vi "Auto.vi"() -> ()   [LabVIEW 2020]
uses:
  Global_Variable/A131258.vi
  Global_Variable/Global.vi
  Database/Global1.vi
  <vilib>/addons/database/Connection.llb/DB Tools Open Connec (String).vi
  <vilib>/addons/database/Connection.llb/Conn Execute.vi
  <vilib>/addons/database/Recordset.llb/Rec Fetch Recordset Data (R).vi
  Global_Variable/A180648.vi
  Libraries/S7/S7.lvlib
  <userlib>/_MGI/1D Array/MGI Running Average/MGI Running Average(DBL[]).vi
  <vilib>/addons/database/NI_Database_API.lvlib
panel:
  out "试验项_Event":refnum<user-event>
  out "标尺_Event":refnum<user-event>
  in  "STEP":string
  out "NVH":bool=TRUE
  out "力特性逆向去程":bool
  out "力特性正向去程":bool
  out "力特性逆向回程":bool
  out "力特性正向回程":bool
  out "逆向空载正向初始化":bool
  out "锁紧/开启初始化":bool
  out "功能正向初始化":bool
  out "功能逆向初始化":bool
  out "空载逆向初始化":bool
  out "空载正向初始化":bool
  out "当前车速":i32
  out "试验项目":T1(tab)
  out "左工位曲线":cluster{dbl[], dbl[]}[](graph)
  out "右工位曲线":cluster{dbl[], dbl[]}[](graph)
  out "角度调节力试验":cluster{dbl[], dbl[]}[](graph)
  out "管柱保持力试验":cluster{dbl[], dbl[]}[](graph)
  out "锁紧/开启":cluster{dbl[], dbl[]}[](graph)
  out "逆向空载试验":cluster{dbl[], dbl[]}[](graph)
  out "振动2NHV-FFT":cluster{"f0":dbl, "df":dbl, "magnitude":dbl[]}[](graph)
  out "振动1NVH-FFT":cluster{"f0":dbl, "df":dbl, "magnitude":dbl[]}[](graph)
  in  "判定结果":bool[][](array[boolean])=[[TRUE]]
  # "."
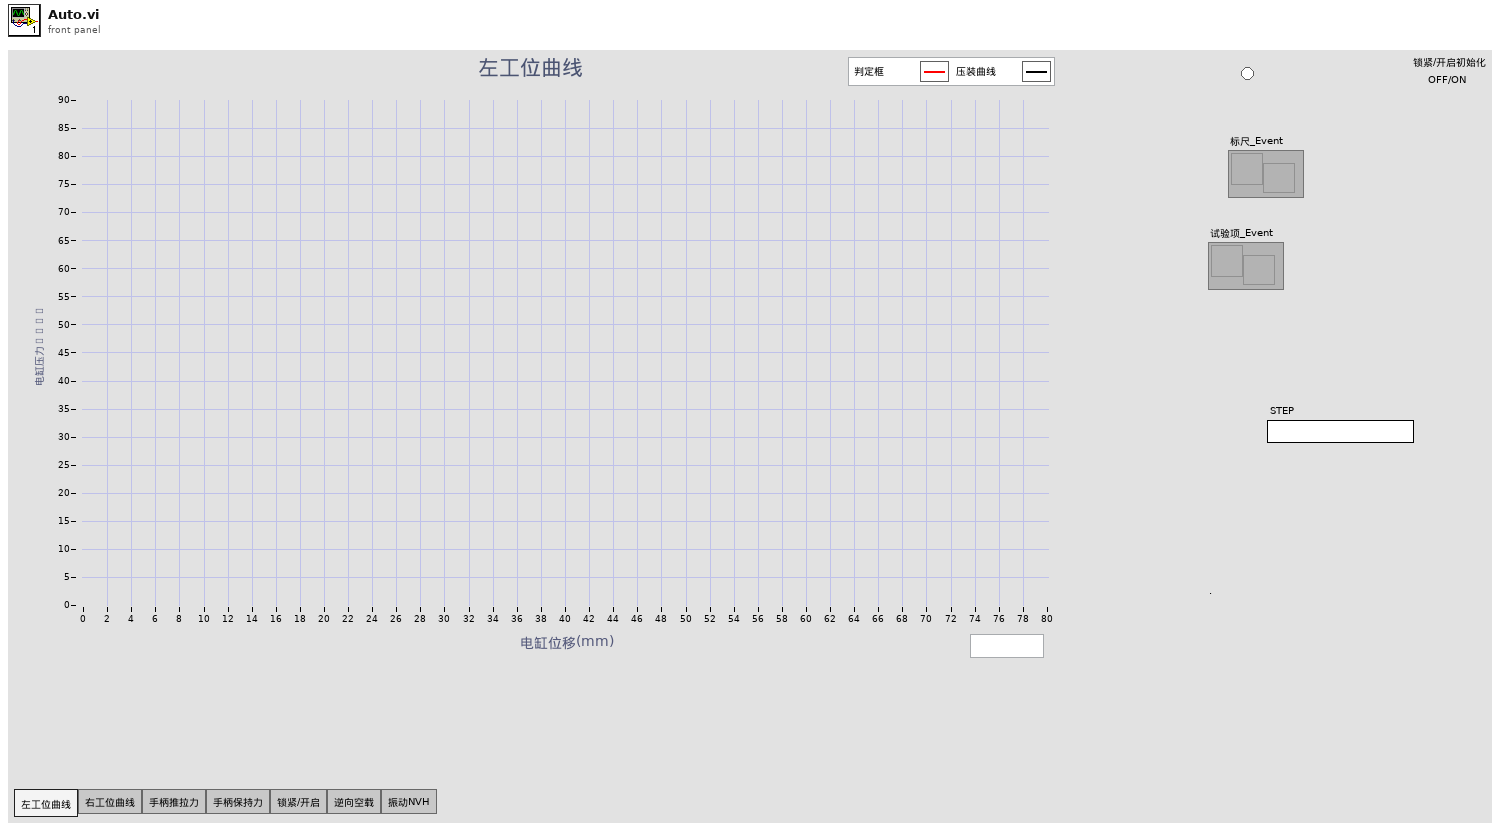
[diagram p1: front panel]
types:
  T1 = enum32{"左工位曲线", "右工位曲线", "手柄推拉力", "手柄保持力", "锁紧/开启", "逆向空载", "振动NVH"}
  T2 = typedef "NI_Database_API.lvlib/Conn ObjectReference.ctl" = refnum<k1>
  T3 = typedef "NI_Database_API.lvlib/Rec ObjectReference.ctl" = refnum<k1>
  T4 = cluster{"左工位最大压力 ":cluster{"单位":string, "下限":dbl, "上限":dbl}, "左工位最小压力":cluster{"单位":string, "下限":dbl, "上限":dbl}, "左工位最终压装位移":cluster{"单位":string, "下限":dbl, "上限":dbl}}
  T5 = cluster{"右工位最大压力 ":cluster{"单位":string, "下限":dbl, "上限":dbl}, "右工位最小压力":cluster{"单位":string, "下限":dbl, "上限":dbl}, "右工位最最终位移":cluster{"单位":string, "下限":dbl, "上限":dbl}}
  T6 = cluster{"X ":cluster{"单位":string, "下限":dbl, "上限":dbl}, "Y":cluster{"单位":string, "下限":dbl, "上限":dbl}}
  T7 = typedef "lveventtype.ctl" = enum32{"Null", "Timeout", "Annotation Menu Selection", "Annotation Menu Selection?", "App Instance Close", "App Instance Close?", "Autoscale Range Change", "Bookmark Info Change", "Cell Edit", "Cell Edit?", "Cursor Grab", "Cursor Grab?", "Cursor Menu Selection", "Cursor Menu Selection?", "Cursor Move", "Cursor Release", "Data Change", "Direction Change", "Display State Change", "Drag Ended", "Drag Enter", "Drag Leave", "Drag Over", "Drag Source Update", "Drag Starting", "Drag Starting?", "Drop", "Exec State Change", "Key Down", "Key Down?", "Key Repeat", "Key Repeat?", "Key Up", "Listbox Double Click", "Menu Activation?", "Menu Selection (App)", "Menu Selection? (App)", "Menu Selection (User)", "Mouse Down", "Mouse Down?", "Mouse Enter", "Mouse Leave", "Mouse Move", "Mouse Up", "Mouse Wheel", "NI Security User Change (App)", "Pane Size", "Panel Close", "Panel Close?", "Panel Resize", "Plot Attribute Change", "Scale Range Change", "Shortcut Menu Activation?", "Shortcut Menu Selection (App)", "Shortcut Menu Selection? (App)", "Shortcut Menu Selection (User)", "Tree Double Click", "Tree Drag", "Tree Drag?", "Tree Drop", "Tree Drop?", "Tree Item Close", "Tree Item Close?", "Tree Item Open", "Tree Item Open?", "User Event", "Value Change"}
  T8 = typedef "LVPoint32TypeDef.ctl" = cluster{"Horizontal":i32, "Vertical":i32}
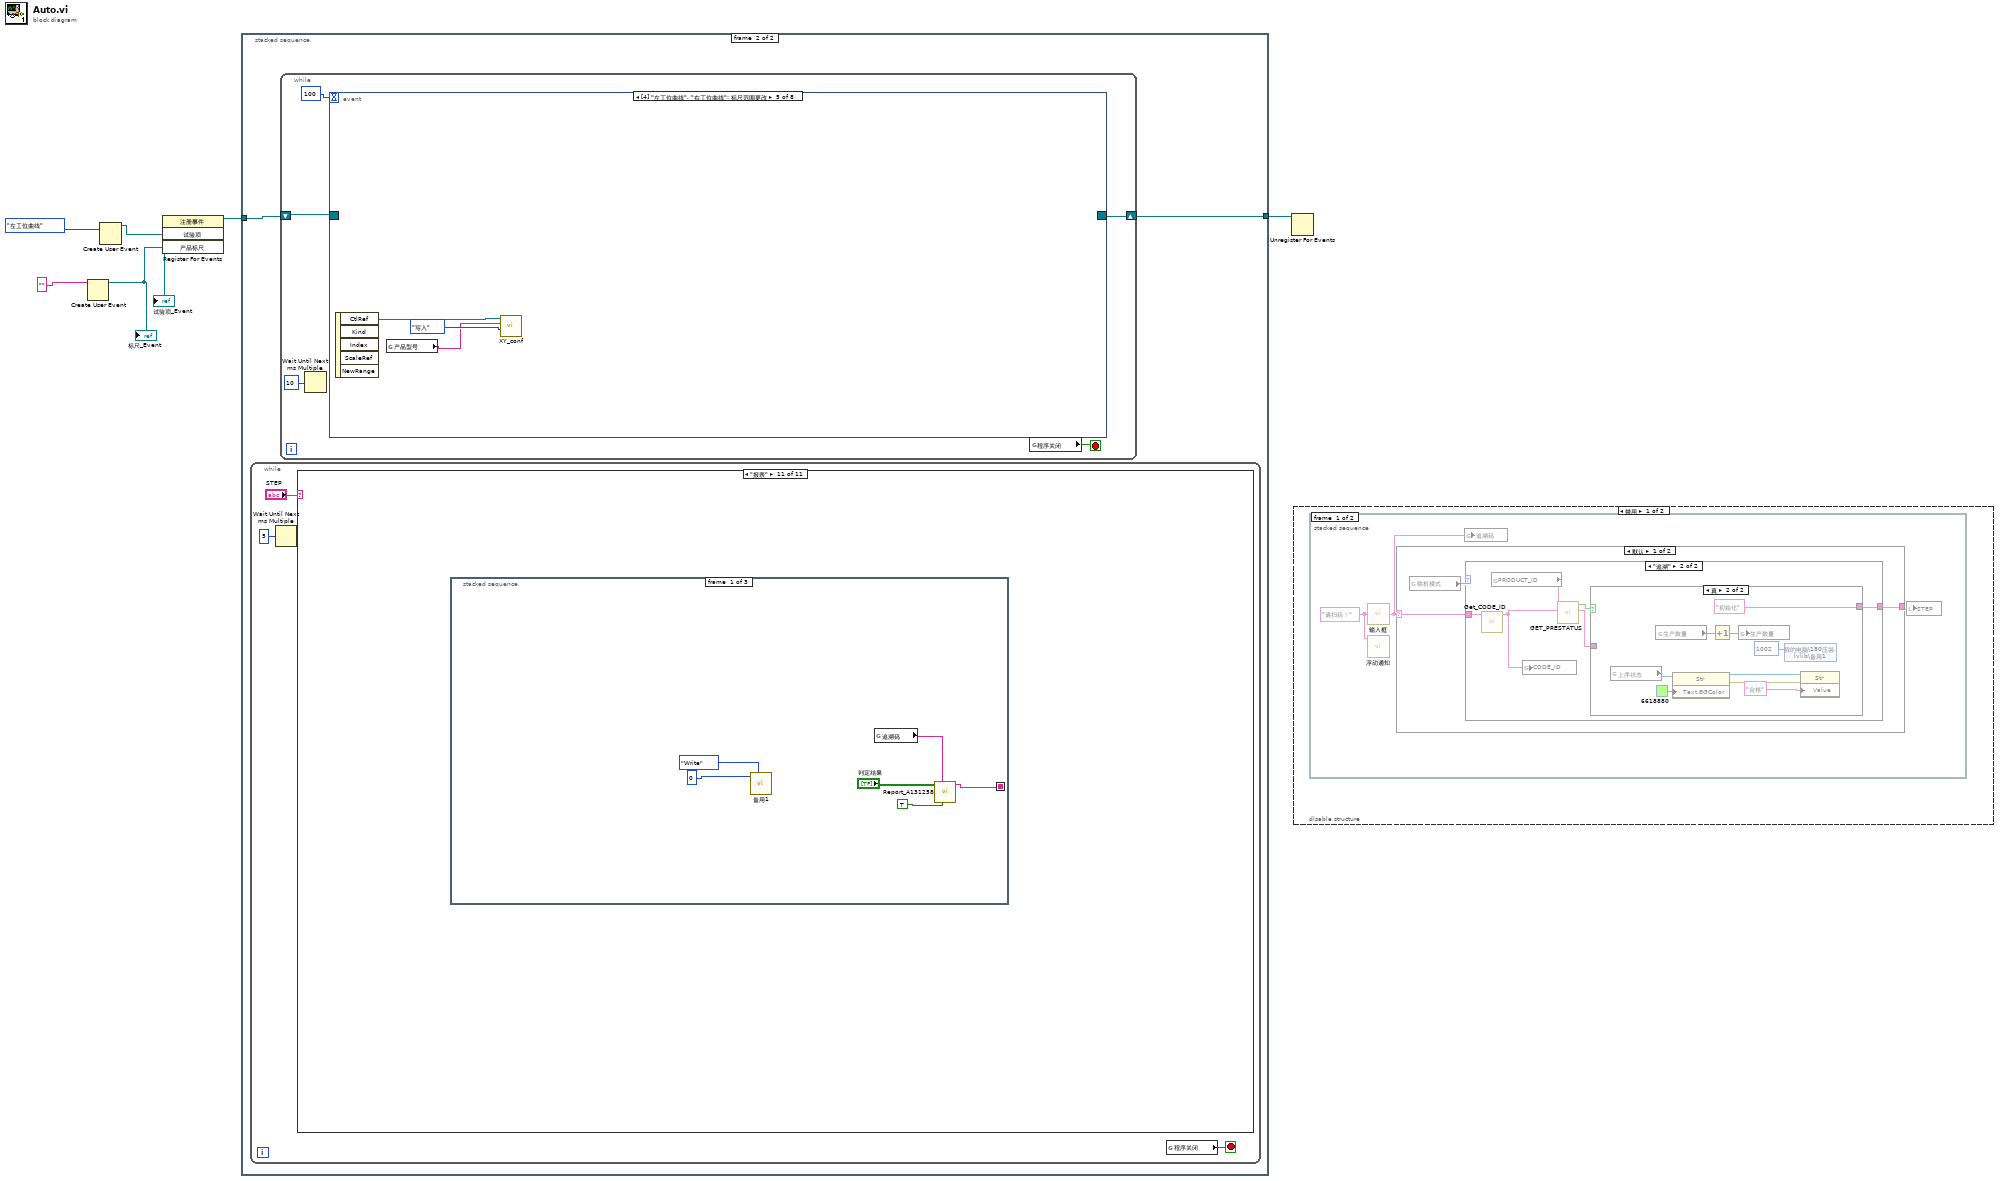
[diagram p0: block diagram]
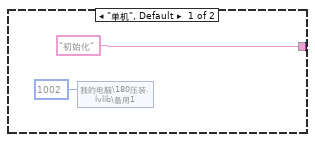
[diagram p2: hidden frame]
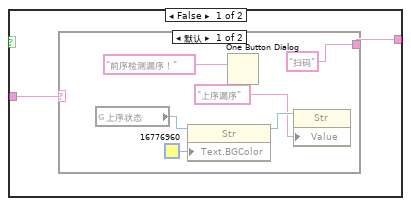
[diagram p3: hidden frame]
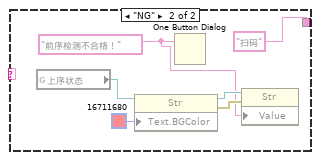
[diagram p4: hidden frame]
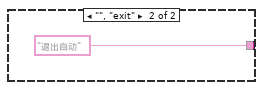
[diagram p5: hidden frame]
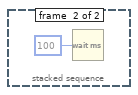
[diagram p6: hidden frame]
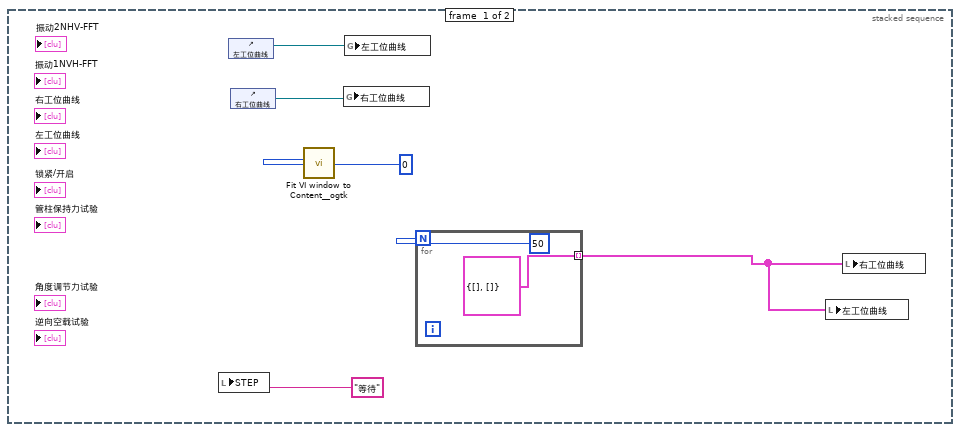
[diagram p8: hidden frame]
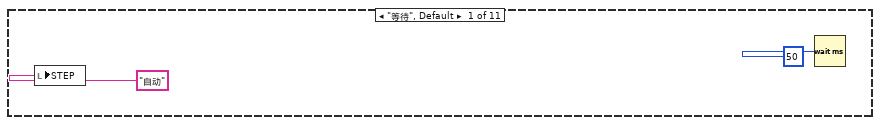
[diagram p9: hidden frame]
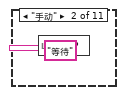
[diagram p10: hidden frame]
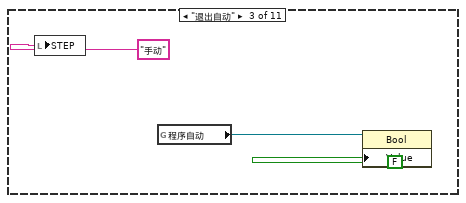
[diagram p11: hidden frame]
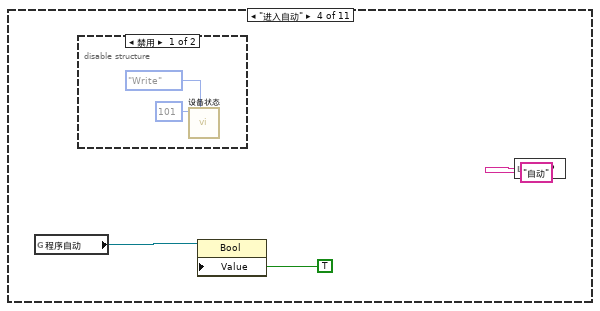
[diagram p12: hidden frame]
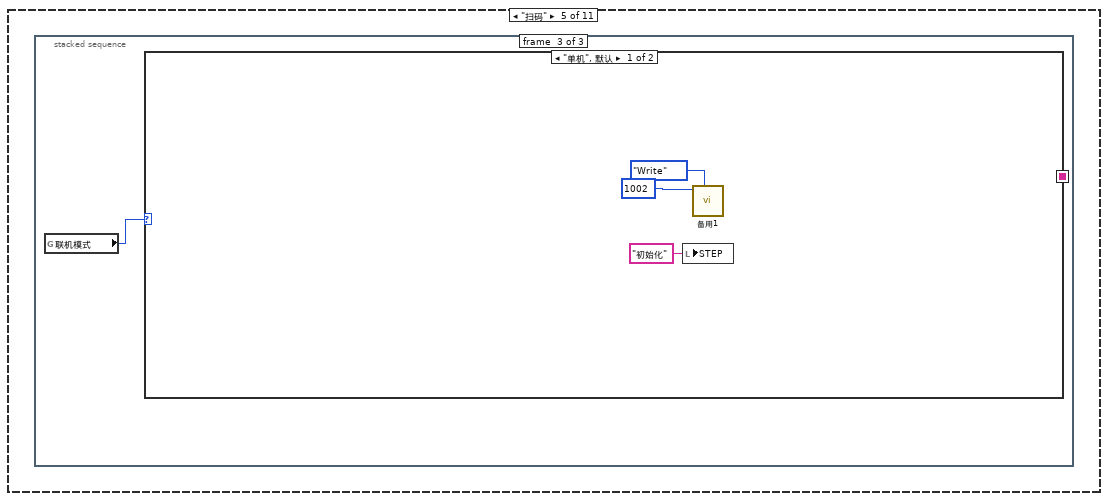
[diagram p14: hidden frame]
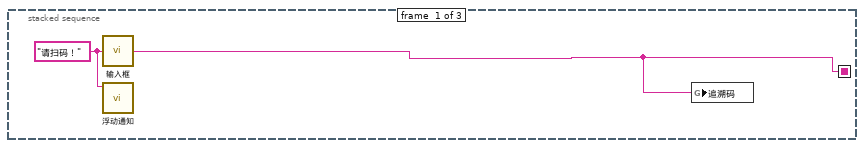
[diagram p15: hidden frame]
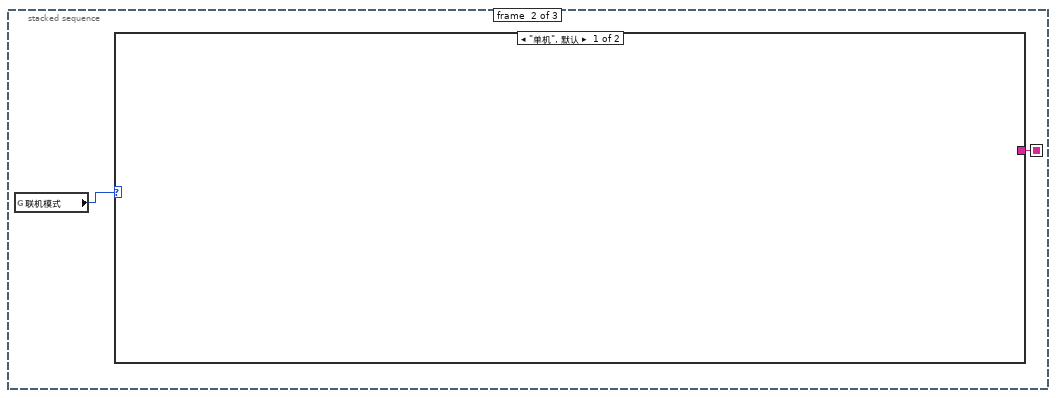
[diagram p16: hidden frame]
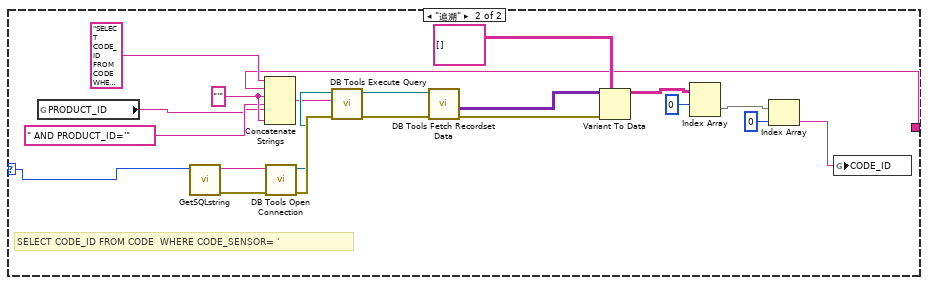
[diagram p17: hidden frame]
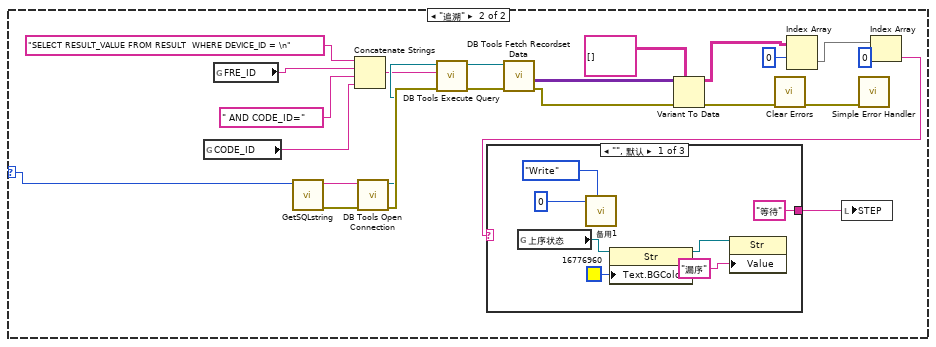
[diagram p18: hidden frame]
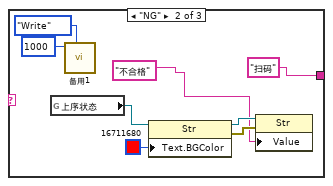
[diagram p19: hidden frame]
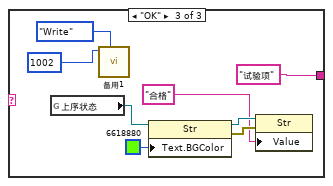
[diagram p20: hidden frame]
diagram:
  n1 = Create User Event(user event datatype="" ("产品标尺")) -> (user event=w4:refnum<user-event>)  [unwired: 1 in, 1 out]
  "标尺_Event" <- w4
  n2 = Create User Event(user event datatype=T1."左工位曲线" ("试验项")) -> (user event=w1:refnum<user-event>)  [unwired: 1 in, 1 out]
  "试验项_Event" <- w1
  n3 = register-events(w1, w4) -> (reference out=w5:refnum<event-registration>)  [unwired: 2 in, 1 out]
  n4 = stacked-sequence {
    tunnel: [_ w15] -> w6
    tunnel: w5 -> [_ w14]
    frame #0 {
      n5 = local write "STEP"("等待" ("STEP")) -> ()
      n6 = control-ref of="左工位曲线"() -> (w11:refnum<vi>)
      n7 = control-ref of="右工位曲线"() -> (w12:refnum<vi>)
      n8 = call "Fit VI window to Content__ogtk.vi"("border spacing (2 px)"=0) -> ()  [unwired: 5 in, 2 out]
      n9 = global write "A131258.vi" "右工位曲线"(w12) -> ()
      n10 = global write "A131258.vi" "左工位曲线"(w11) -> ()
      n11 = for {
        N: 50 -> [_]
        tunnel: [cluster{dbl[], dbl[]} {[], []}] -> w8 mode=indexing
      }
      n12 = local write "左工位曲线"(w8) -> ()
      n13 = local write "右工位曲线"(w8) -> ()
    }
    frame #1 {
      n14 = while {
        stop <- w18 stop-if-true
        n15 = Wait Until Next ms Multiple(millisecond multiple=u32 5 ("毫秒倍数")) -> ()  [unwired: 1 out]
        n16 = case shown="\"报表\"" "STEP" {
          frame "等待", Default {
            n17 = local write "STEP"("自动" ("STEP")) -> ()
            n18 = Wait (ms)(milliseconds to wait=u32 50 ("等待时间（毫秒）")) -> ()  [unwired: 1 out]
          }
          frame "手动" {
            n19 = local write "STEP"("等待" ("STEP")) -> ()
          }
          frame "退出自动" {
            n20 = local write "STEP"("手动" ("STEP")) -> ()
            n21 = global read "Global.vi" "程序自动"() -> (w23:refnum<vi>)
            n22 = property class="Bool"(reference=w23, "Value"=FALSE) -> ()  [unwired: 1 in, 2 out]
          }
          frame "进入自动" {
            n23 = global read "Global.vi" "程序自动"() -> (w26:refnum<vi>)
            n24 = disable-structure shown="禁用" {
              frame Disabled {
                n25 = call "设备状态.vi"("枚举"=enum16{"Read", "Write"}."Write", "Status_Write"=i16 101) -> ()  [unwired: 9 in, 1 out]
              }
              frame Enabled {
              }
            }
            n26 = property class="Bool"(reference=w26, "Value"=TRUE) -> ()  [unwired: 1 in, 2 out]
            n27 = local write "STEP"("自动" ("STEP")) -> ()
          }
          frame "扫码" {
            n28 = stacked-sequence {
              seq-local: [w30 _ _] -> [_ w33 _]
              frame #0 {
                w31 = "请扫码！" ("提示信息")
                n29 = call "输入框.vi"("提示信息"=w31) -> ("条形码输出"=w30:string)
                n30 = call "浮动通知.vi"("通知内容"=w31) -> ()  [unwired: 11 in]
                n31 = global write "Global.vi" "追溯码"(w30) -> ()
              }
              frame #1 {
                n32 = global read "Global1.vi" "联机模式"() -> (w32:enum16{"单机", "追溯"})
                n33 = case shown="\"单机\", 默认" w32 {
                  selector: w32 -> [_ w34]
                  tunnel: w33 -> [_ w37]
                  frame "单机", Default {
                  }
                  frame "追溯" {
                    w54 = "'" ("字符串")
                    # "SELECT CODE_ID FROM CODE  WHERE CODE_SENSOR= '"
                    n34 = global read "Global.vi" "PRODUCT_ID"() -> (w36:string)
                    n35 = call "GetSQLstring.vi"("联机模式"=w34) -> ("错误输出"=w40:errorcluster, "连接字符串"=w39:string)  [unwired: 9 in]
                    n36 = Concatenate Strings("SELECT CODE_ID FROM CODE  WHERE CODE_MAIN= '" ("table"), w37, w54, " AND PRODUCT_ID='" ("字符串"), w36, w54) -> (w41:string)
                    n37 = call-poly <vilib>:"DB Tools Open Connection.vi"("error in (no error)"=w40, "connection information"=w39) -> ("error out"=w46:errorcluster, "connection reference"=w45:T2)  [unwired: 6 in]
                    n38 = call-poly <vilib>:"DB Tools Execute Query.vi"("error in (no error)"=w46, "SQL query"=w41, "connection reference"=w45) -> ("error out"=w43:errorcluster, "recordset reference"=w42:T3)  [unwired: 5 in]
                    n39 = call-poly <vilib>:"DB Tools Fetch Recordset Data.vi"("error in (no error)"=w43, "recordset reference"=w42) -> ("error out"=w48:errorcluster, "recordset data"=w44:variant[][])  [unwired: 3 in, 1 out]
                    n40 = Variant To Data(error in=w48, type=string[][] [], Variant=w44) -> (data=w49:string[][])  [unwired: 1 out]
                    n41 = Index Array(array=w49, index (row)=0 ("索引 (行)")) -> (element=w51:string[])  [unwired: 1 in]
                    n42 = Index Array(array=w51, index=0 ("索引 (行)")) -> (element=w35:string)
                    n43 = global write "Global.vi" "CODE_ID"(w35) -> ()
                  }
                }
              }
              frame #2 {
                n44 = global read "Global1.vi" "联机模式"() -> (w55:enum16{"单机", "追溯"})
                n45 = case shown="\"单机\", 默认" w55 {
                  selector: w55 -> [_ w59]
                  frame "单机", Default {
                    n46 = local write "STEP"("初始化" ("STEP")) -> ()
                    n47 = call "备用1.vi"("枚举"=enum16{"Read", "Write"}."Write", "Status_Write"=u16 1002 ("备用1")) -> ()  [unwired: 9 in, 1 out]
                  }
                  frame "追溯" {
                    n48 = global read "Global.vi" "CODE_ID"() -> (w62:string)
                    n49 = global read "Global.vi" "FRE_ID"() -> (w63:string)
                    n50 = call "GetSQLstring.vi"("联机模式"=w59) -> ("错误输出"=w65:errorcluster, "连接字符串"=w64:string)  [unwired: 9 in]
                    n51 = Concatenate Strings("SELECT RESULT_VALUE FROM RESULT  WHERE DEVICE_ID = \n" ("table"), w63, " AND CODE_ID=" ("字符串"), w62) -> (w66:string)
                    n52 = call-poly <vilib>:"DB Tools Open Connection.vi"("error in (no error)"=w65, "connection information"=w64) -> ("error out"=w72:errorcluster, "connection reference"=w71:T2)  [unwired: 6 in]
                    n53 = call-poly <vilib>:"DB Tools Execute Query.vi"("error in (no error)"=w72, "SQL query"=w66, "connection reference"=w71) -> ("error out"=w68:errorcluster, "recordset reference"=w67:T3)  [unwired: 5 in]
                    n54 = call-poly <vilib>:"DB Tools Fetch Recordset Data.vi"("error in (no error)"=w68, "recordset reference"=w67) -> ("error out"=w74:errorcluster, "recordset data"=w69:variant[][])  [unwired: 3 in, 1 out]
                    n55 = Variant To Data(error in=w74, type=string[][] [], Variant=w69) -> (data=w78:string[][], error out=w79:errorcluster)
                    n56 = call <vilib>:"Clear Errors.vi"("error in (no error)"=w79) -> ("error out"=w80:errorcluster)  [unwired: 5 in, 1 out]
                    n57 = Index Array(array=w78, index (row)=0 ("索引 (行)")) -> (element=w76:string[])  [unwired: 1 in]
                    n58 = call <vilib>:"Simple Error Handler.vi"("error in (no error)"=w80) -> ()  [unwired: 4 in, 5 out]
                    n59 = Index Array(array=w76, index=0 ("索引 (行)")) -> (element=w61:string)
                    n60 = case shown="\"\", 默认" w61 {
                      tunnel: ["等待" ("State(s) in Front (\"\")") "扫码" ("State(s) in Front (\"\")") "试验项" ("State(s) in Front (\"\")")] -> w60
                      frame "", Default {
                        n61 = global read "Global.vi" "上序状态"() -> (w85:refnum<vi>)
                        n62 = call "备用1.vi"("枚举"=enum16{"Read", "Write"}."Write", "Status_Write"=u16 0 ("备用1")) -> ()  [unwired: 9 in, 1 out]
                        n63 = property class="Str"(reference=w85, "Text.BGColor"=u32 16776960 ("文本.文本颜色:背景色")) -> (reference out=w86:refnum<vi>)  [unwired: 1 in, 1 out]
                        n64 = property class="Str"(reference=w86, "Value"="漏序" ("上序状态")) -> ()  [unwired: 1 in, 2 out]
                      }
                      frame "NG" {
                        n65 = global read "Global.vi" "上序状态"() -> (w92:refnum<vi>)
                        n66 = call "备用1.vi"("枚举"=enum16{"Read", "Write"}."Write", "Status_Write"=i16 1000) -> ()  [unwired: 9 in, 1 out]
                        n67 = property class="Str"(reference=w92, "Text.BGColor"=u32 16711680 ("文本.文本颜色:背景色")) -> (reference out=w95:refnum<vi>, error out=w94:errorcluster)  [unwired: 1 in]
                        n68 = property class="Str"(reference=w95, error in=w94, "Value"="不合格" ("消息")) -> ()  [unwired: 2 out]
                      }
                      frame "OK" {
                        n69 = global read "Global.vi" "上序状态"() -> (w100:refnum<vi>)
                        n70 = call "备用1.vi"("枚举"=enum16{"Read", "Write"}."Write", "Status_Write"=u16 1002 ("备用1")) -> ()  [unwired: 9 in, 1 out]
                        n71 = property class="Str"(reference=w100, "Text.BGColor"=u32 6618880 ("文本.文本颜色:背景色")) -> (reference out=w103:refnum<vi>, error out=w102:errorcluster)  [unwired: 1 in]
                        n72 = property class="Str"(reference=w103, error in=w102, "Value"="合格" ("消息")) -> ()  [unwired: 2 out]
                      }
                    }
                    n73 = local write "STEP"(w60) -> ()
                  }
                }
              }
            }
          }
          frame "等待启动" {
            n74 = local write "STEP"("等待" ("STEP")) -> ()
          }
          frame "初始化" {
            n75 = stacked-sequence {
              frame #0 {
                w106 = 0 ("当前车速")
                n76 = local write "判定结果"(bool[][] [] ("判定结果")) -> ()
                n77 = global write "Global.vi" "右判定长度"(w106) -> ()
                n78 = global write "Global.vi" "左判定长度"(w106) -> ()
                "当前车速" <- w106
              }
              frame #1 {
                w111 = TRUE
                n79 = global read "Global.vi" "试验项目"() -> (w110:bool[])
                n80 = Index Array(array=w110, index=4 ("索引")) -> (element=w108:bool)
                n81 = case shown="假" w108 {
                  frame False {
                    n82 = local write "锁紧/开启初始化"(FALSE ("锁紧/开启初始化")) -> ()
                  }
                  frame True {
                    "锁紧/开启初始化" <- TRUE ("锁紧/开启初始化")
                  }
                }
                "逆向空载正向初始化" <- w111
                "空载正向初始化" <- w111
                "空载逆向初始化" <- w111
                "功能正向初始化" <- w111
                "功能逆向初始化" <- w111
                "力特性逆向去程" <- w111
                "力特性正向去程" <- w111
                "力特性逆向回程" <- w111
                "力特性正向回程" <- w111
              }
              frame #2 {
                n83 = for {
                  N: 50 -> [_]
                  tunnel: [cluster{dbl[], dbl[]} {[], []}] -> w115 mode=indexing
                  tunnel: [cluster{"f0":dbl, "df":dbl, "magnitude":dbl[]} {"f0"=0.0, "df"=0.0, "magnitude"=[]} ("power spectrum [dB EU]")] -> w114 mode=indexing
                }
                n84 = local write "角度调节力试验"(w115) -> ()
                n85 = local write "管柱保持力试验"(w115) -> ()
                n86 = local write "逆向空载试验"(w115) -> ()
                n87 = local write "锁紧/开启"(w115) -> ()
                n88 = local write "左工位曲线"(w115) -> ()
                n89 = local write "右工位曲线"(w115) -> ()
                n90 = local write "振动2NHV-FFT"(w114) -> ()
                n91 = local write "振动1NVH-FFT"(w114) -> ()
              }
              frame #3 {
                w120 = -2
                n92 = global read "Global.vi" "Result"() -> (w122:refnum<vi>)
                n93 = Bundle(w120, w120) -> (w119:cluster{i32, i32})  [unwired: 1 in]
                n94 = property class="Tbl"(reference=w122, "Value"=string[][] []) -> (reference out=w125:refnum<vi>, error out=w126:errorcluster)  [unwired: 1 in]
                n95 = property class="Tbl"(reference=w122, "Active Cell"=w119, "Cell BG Color"=u32 16777216 ("活动单元格:单元格背景色")) -> ()  [unwired: 1 in, 2 out]
                n96 = property class="Tbl"(reference=w125, error in=w126, "Row Headers[]"=string[] [] ("列首字符串[]")) -> ()  [unwired: 2 out]
              }
              frame #4 {
                n97 = global read "A131258.vi" "LED-左工位"() -> (w128:refnum<vi>)
                n98 = global read "A131258.vi" "LED-右工位"() -> (w127:refnum<vi>)
                n99 = Build Array(w128, w127) -> (w129:refnum<vi>[])
                n100 = for {
                  tunnel: w129 -> [w130] mode=indexing
                  n101 = property class="Bool"(reference=w130, "Colors [4]"=cluster{u32, u32}[] [{12369084, 12369084}] ("颜色[4]")) -> ()  [unwired: 1 in, 2 out]
                }
              }
              frame #5 {
                n102 = global write "Global.vi" "当前试验项"(enum16{"左工位", "右工位", "完成"}."左工位" ("当前试验项")) -> ()
                n103 = local write "STEP"("试验项" ("STEP")) -> ()
              }
            }
          }
          frame "试验项" {
            n104 = global read "Global.vi" "当前试验项"() -> (w134:enum16{"左工位", "右工位", "完成"})
            n105 = case shown="\"完成\"" w134 {
              selector: w134 -> [w136 _]
              tunnel: [w139 "报表" ("STEP")] -> w135
              frame "左工位", Default {
                n106 = global read "Global.vi" "试验项目"() -> (w137:bool[])
                n107 = Index Array(array=w137, index=w136) -> (element=w138:bool)
                n108 = case shown="真" w138 {
                  selector: w138 -> [_ w146]
                  tunnel: ["试验项" ("字符串") w147] -> w139
                  tunnel: w136 -> [_ w148]
                  frame False {
                    n109 = global read "Global.vi" "当前试验项"() -> (w141:enum16{"左工位", "右工位", "完成"})
                    n110 = Increment(x=w141) -> (x+1=w140:enum16{"左工位", "右工位", "完成"})
                    n111 = local read "判定结果"() -> (w142:bool[][])
                    n112 = global write "Global.vi" "当前试验项"(w140) -> ()
                    n113 = Build Array (concatenate)(w142, bool[] [FALSE] ("判定结果")) -> (w143:bool[][])
                    n114 = local write "判定结果"(w143) -> ()
                  }
                  frame True {
                    n115 = case shown="\"右工位\"" w148 {
                      tunnel: [w163 "等待" ("STEP") "试验项" ("STEP")] -> w147
                      tunnel: w146 -> [_ _ _]
                      frame "左工位", Default {
                        w156 = -2
                        n116 = global read "Global.vi" "Result"() -> (w158:refnum<vi>)
                        n117 = global write "Global.vi" "左判定长度"(0 ("左判定长度")) -> ()
                        n118 = property class="Tbl"(reference=w158, "Value"=string[][] []) -> (reference out=w161:refnum<vi>, error out=w162:errorcluster)  [unwired: 1 in]
                        n119 = local write "判定结果"(bool[][] [[FALSE]] ("判定结果")) -> ()
                        n120 = Bundle(w156, w156) -> (w155:cluster{i32, i32})  [unwired: 1 in]
                        n121 = global read "Global.vi" "复选框"() -> (w149:bool)
                        n122 = property class="Tbl"(reference=w161, error in=w162, "Row Headers[]"=string[] [] ("列首字符串[]")) -> ()  [unwired: 2 out]
                        n123 = property class="Tbl"(reference=w158, "Active Cell"=w155, "Cell BG Color"=u32 16777216 ("活动单元格:单元格背景色")) -> ()  [unwired: 1 in, 2 out]
                        n124 = global read "A131258.vi" "LED-右工位"() -> (w153:refnum<vi>)
                        n125 = global read "A131258.vi" "LED-左工位"() -> (w154:refnum<vi>)
                        n126 = case shown="假" w149 {
                          tunnel: ["试验项" ("STEP") "等待" ("STEP")] -> w163
                          frame False {
                            n127 = global read "Global.vi" "当前试验项"() -> (w165:enum16{"左工位", "右工位", "完成"})
                            n128 = Increment(x=w165) -> (x+1=w164:enum16{"左工位", "右工位", "完成"})
                            n129 = global write "Global.vi" "当前试验项"(w164) -> ()
                          }
                          frame True {
                            n130 = property on="试验项目" class="TabCtl (严格)"("Val(Sgnl)"=T1."左工位曲线" ("值(信号)")) -> ()  [unwired: 2 in, 2 out]
                            n131 = call "浮动通知.vi"("通知内容"="左工位压装") -> ()  [unwired: 11 in]
                          }
                        }
                        n132 = Build Array(w154, w153) -> (w152:refnum<vi>[])
                        n133 = for {
                          tunnel: w152 -> [w171] mode=indexing
                          n134 = property class="Bool"(reference=w171, "Colors [4]"=cluster{u32, u32}[] [{12369084, 12369084}] ("颜色[4]")) -> ()  [unwired: 1 in, 2 out]
                        }
                      }
                      frame "右工位" {
                        n135 = global read "Global.vi" "试验项目"() -> (w174:bool[])
                        n136 = property on="试验项目" class="TabCtl (严格)"("Val(Sgnl)"=T1."右工位曲线" ("值(信号)")) -> ()  [unwired: 2 in, 2 out]
                        n137 = call "浮动通知.vi"("通知内容"="右工位压装") -> ()  [unwired: 11 in]
                        n138 = Index Array(array=w174, index=0 ("索引")) -> (element=w173:bool)
                        n139 = case shown="假" w173 {
                          frame False {
                            w184 = -2
                            n140 = global read "Global.vi" "Result"() -> (w186:refnum<vi>)
                            n141 = Bundle(w184, w184) -> (w183:cluster{i32, i32})  [unwired: 1 in]
                            n142 = global write "Global.vi" "左判定长度"(0 ("左判定长度")) -> ()
                            n143 = property class="Tbl"(reference=w186, "Value"=string[][] []) -> (reference out=w189:refnum<vi>, error out=w190:errorcluster)  [unwired: 1 in]
                            n144 = property class="Tbl"(reference=w186, "Active Cell"=w183, "Cell BG Color"=u32 16777216 ("活动单元格:单元格背景色")) -> ()  [unwired: 1 in, 2 out]
                            n145 = property class="Tbl"(reference=w189, error in=w190, "Row Headers[]"=string[] [] ("列首字符串[]")) -> ()  [unwired: 2 out]
                            n146 = global read "A131258.vi" "LED-右工位"() -> (w181:refnum<vi>)
                            n147 = global read "A131258.vi" "LED-左工位"() -> (w182:refnum<vi>)
                            n148 = local write "判定结果"(bool[][] [[FALSE]] ("判定结果")) -> ()
                            n149 = Build Array(w182, w181) -> (w180:refnum<vi>[])
                            n150 = for {
                              tunnel: w180 -> [w192] mode=indexing
                              n151 = property class="Bool"(reference=w192, "Colors [4]"=cluster{u32, u32}[] [{12369084, 12369084}] ("颜色[4]")) -> ()  [unwired: 1 in, 2 out]
                            }
                          }
                          frame True {
                          }
                        }
                      }
                      frame "完成" {
                        n152 = call "浮动通知.vi"("通知内容"="压装完成") -> ()  [unwired: 11 in]
                      }
                    }
                  }
                }
              }
              frame "完成" {
                n153 = Wait (ms)(milliseconds to wait=u32 200 ("等待时间（毫秒）")) -> ()  [unwired: 1 out]
              }
            }
            n154 = local write "STEP"(w135) -> ()
          }
          frame "判定" {
            n155 = stacked-sequence {
              frame #0 {
                n156 = global read "Global.vi" "当前试验项"() -> (w197:enum16{"左工位", "右工位", "完成"})
                n157 = case shown="\"左工位\"" w197 {
                  frame "完成", Default {
                  }
                  frame "左工位" {
                    n158 = global read "Global.vi" "左工位判定参数"() -> (w200:T4)
                    n159 = global read "A131258.vi" "LED-左工位"() -> (w198:refnum<vi>)
                    n160 = local read "左工位曲线"() -> (w210:cluster{dbl[], dbl[]}[])
                    n161 = global read "Global.vi" "Result"() -> (w209:refnum<vi>)
                    n162 = call "左工位判定.vi"("Result"=w209, "左工位判定"=w200, "XY曲线"=w210) -> ("大小"=w199:i32, "OK？"=w201:bool)  [unwired: 7 in]
                    n163 = Select(t=cluster{u32, u32}[] [{6618880, 6618880}, {6618880, 6618880}, {6618880, 6618880}, {6618880, 6618880}] ("颜色[4]"), s=w201, f=cluster{u32, u32}[] [{16711680, 16711680}, {16711680, 16711680}, {16711680, 16711680}, {16711680, 16711680}] ("颜色[4]")) -> (s? t:f=w206:cluster{u32, u32}[])
                    n164 = property class="Bool"(reference=w198, "Colors [4]"=w206) -> ()  [unwired: 1 in, 2 out]
                    n165 = local read "判定结果"() -> (w202:bool[][])
                    n166 = case shown="假" w201 {
                      frame False {
                        w211 = 4 items=["OK", "OKCancel", "AbortRetryIgnore", "YesNoCancel", "YesNo", "RetryCancel"] ("buttons")
                        w213 = 64 items=["None"=0, "Hand, Error, Stop"=16, "Question"=32, "Exclamation, Warning"=48, "Asterisk, Information"=64] ("icon")
                        n167 = call "信息框（标题、文本、图标）.vi"("icon"=w213, "buttons"=w211, "caption"="不合格", "text"="压装不合格是否进行下工位压装" ("消息")) -> ("按钮输出"=w212:i32)  [unwired: 6 in, 1 out]
                        n168 = case shown="7" w212 {
                          frame 6, Default {
                            n169 = local write "STEP"("报表" ("STEP")) -> ()
                          }
                          frame 7 {
                            n170 = global read "Global.vi" "当前试验项"() -> (w219:enum16{"左工位", "右工位", "完成"})
                            n171 = Increment(x=w219) -> (x+1=w220:enum16{"左工位", "右工位", "完成"})
                            n172 = global write "Global.vi" "当前试验项"(w220) -> ()
                          }
                        }
                        n173 = call "合格状态.vi"("枚举"=enum16{"Read", "Write"}."Write", "Status_Write"=i16 2) -> ()  [unwired: 9 in, 1 out]
                      }
                      frame True {
                        n174 = call "合格状态.vi"("枚举"=enum16{"Read", "Write"}."Write", "Status_Write"=i16 1) -> ()  [unwired: 9 in, 1 out]
                      }
                    }
                    n175 = Build Array(TRUE, w201) -> (w205:bool[])
                    n176 = Build Array (concatenate)(w202, w205) -> (w203:bool[][])
                    n177 = local write "判定结果"(w203) -> ()
                    n178 = global write "Global.vi" "左判定长度"(w199) -> ()
                  }
                  frame "右工位" {
                    n179 = global read "Global.vi" "右工位判定参数"() -> (w223:T5)
                    n180 = local read "右工位曲线"() -> (w236:cluster{dbl[], dbl[]}[])
                    n181 = global read "A131258.vi" "LED-右工位"() -> (w225:refnum<vi>)
                    n182 = global read "Global.vi" "Result"() -> (w235:refnum<vi>)
                    n183 = call "右工位判定.vi"("Result"=w235, "右工位判定"=w223, "XY曲线"=w236) -> ("大小"=w224:i32, "OK？"=w226:bool)  [unwired: 7 in]
                    n184 = Select(t=cluster{u32, u32}[] [{6618880, 6618880}, {6618880, 6618880}, {6618880, 6618880}, {6618880, 6618880}] ("颜色[4]"), s=w226, f=cluster{u32, u32}[] [{16711680, 16711680}, {16711680, 16711680}, {16711680, 16711680}, {16711680, 16711680}] ("颜色[4]")) -> (s? t:f=w232:cluster{u32, u32}[])
                    n185 = property class="Bool"(reference=w225, "Colors [4]"=w232) -> ()  [unwired: 1 in, 2 out]
                    n186 = local read "判定结果"() -> (w228:bool[][])
                    n187 = Build Array(TRUE, w226) -> (w231:bool[])
                    n188 = global write "Global.vi" "右判定长度"(w224) -> ()
                    n189 = Build Array (concatenate)(w228, w231) -> (w229:bool[][])
                    n190 = case shown="真" w226 {
                      frame False {
                        n191 = call "合格状态.vi"("枚举"=enum16{"Read", "Write"}."Write", "Status_Write"=i16 2) -> ()  [unwired: 9 in, 1 out]
                      }
                      frame True {
                        n192 = call "合格状态.vi"("枚举"=enum16{"Read", "Write"}."Write", "Status_Write"=i16 1) -> ()  [unwired: 9 in, 1 out]
                      }
                    }
                    n193 = local write "判定结果"(w229) -> ()
                    "NVH" <- TRUE
                  }
                }
              }
              frame #1 {
                n194 = global read "Global.vi" "当前试验项"() -> (w243:enum16{"左工位", "右工位", "完成"})
                n195 = Increment(x=w243) -> (x+1=w242:enum16{"左工位", "右工位", "完成"})
                n196 = local write "STEP"("试验项" ("STEP")) -> ()
                n197 = Wait (ms)(milliseconds to wait=u32 500 ("等待时间（毫秒）")) -> ()  [unwired: 1 out]
                n198 = global write "Global.vi" "当前试验项"(w242) -> ()
              }
            }
          }
          frame "自动" {
            n199 = call "备用1.vi"("枚举"=enum16{"Read", "Write"}."Read") -> ("Status_Read"=w246:i16)  [unwired: 10 in]
            n200 = case shown="1000" w246 {
              frame 0, Default {
              }
              frame 1 {
                n201 = call "备用2.vi"("枚举"=enum16{"Read", "Write"}."Read") -> ("Status_Read"=w250:i16)  [unwired: 10 in]
                n202 = call "传感器数据.vi"() -> ("电缸位移"=w248:sgl, "电缸自带压力"=w247:sgl)  [unwired: 7 in, 3 out]
                n203 = case shown="2" w250 {
                  tunnel: w248 -> [_ w252 w261]
                  tunnel: w247 -> [_ w251 w260]
                  frame 0, Default {
                  }
                  frame 1 {
                    n204 = control-ref of="左工位曲线"() -> (w256:refnum<vi>)
                    n205 = call "曲线采集.vi"("曲线引用"=w256, "曲线索引"=1, "X"=w252, "Y"=w251) -> ("错误输出"=w254:errorcluster)  [unwired: 10 in, 1 out]
                    n206 = Unbundle By Name(w254) -> ("status"=w253:bool)
                    n207 = local read "空载正向初始化"() -> (w257:bool)
                    n208 = local write "空载正向初始化"(w253) -> ()
                    n209 = disable-structure shown="禁用" {
                      disable-tunnel: w257 -> [w259 _]
                      frame Disabled {
                        w258 = 2 ("Averaging Size")
                        n210 = call-poly <userlib>:"MGI Running Average.vi"("Averaging Size"=w258, "Initialize? (F)"=w259) -> ()  [unwired: 9 in, 1 out]
                        n211 = call-poly <userlib>:"MGI Running Average.vi"("Averaging Size"=w258, "Initialize? (F)"=w259) -> ()  [unwired: 9 in, 1 out]
                      }
                      frame Enabled {
                      }
                    }
                  }
                  frame 2 {
                    n212 = control-ref of="右工位曲线"() -> (w265:refnum<vi>)
                    n213 = call "曲线采集.vi"("曲线引用"=w265, "曲线索引"=1, "X"=w261, "Y"=w260) -> ("错误输出"=w263:errorcluster)  [unwired: 10 in, 1 out]
                    n214 = Unbundle By Name(w263) -> ("status"=w262:bool)
                    n215 = local read "空载正向初始化"() -> (w266:bool)
                    n216 = local write "空载正向初始化"(w262) -> ()
                    n217 = disable-structure shown="禁用" {
                      disable-tunnel: w266 -> [w268 _]
                      frame Disabled {
                        w267 = 2 ("Averaging Size")
                        n218 = call-poly <userlib>:"MGI Running Average.vi"("Averaging Size"=w267, "Initialize? (F)"=w268) -> ()  [unwired: 9 in, 1 out]
                        n219 = call-poly <userlib>:"MGI Running Average.vi"("Averaging Size"=w267, "Initialize? (F)"=w268) -> ()  [unwired: 9 in, 1 out]
                      }
                      frame Enabled {
                      }
                    }
                  }
                }
              }
              frame 2 {
                n220 = flat-sequence {
                  frame #0 {
                    n221 = Wait (ms)(milliseconds to wait=u32 50 ("等待时间（毫秒）")) -> ()  [unwired: 1 out]
                    n222 = call "备用1.vi"("枚举"=enum16{"Read", "Write"}."Write", "Status_Write"=u16 0 ("备用1")) -> ()  [unwired: 9 in, 1 out]
                  }
                  frame #1 {
                    n223 = local write "STEP"("判定" ("STEP")) -> ()
                  }
                }
              }
              frame 3 {
                n224 = local write "STEP"("判定" ("STEP")) -> ()
                n225 = call "备用1.vi"("枚举"=enum16{"Read", "Write"}."Write", "Status_Write"=u16 0 ("备用1")) -> ()  [unwired: 9 in, 1 out]
              }
              frame 100 {
                n226 = global read "Global.vi" "当前试验项"() -> (w276:enum16{"左工位", "右工位", "完成"})
                n227 = case shown="\"左工位\"" w276 {
                  frame "完成", Default {
                  }
                  frame "左工位" {
                    n228 = stacked-sequence {
                      frame #0 {
                        n229 = for {
                          N: 50 -> [_]
                          tunnel: [cluster{dbl[], dbl[]} {[], []}] -> w277 mode=indexing
                        }
                        n230 = local write "左工位曲线"(w277) -> ()
                      }
                      frame #1 {
                        n231 = local read "左工位曲线"() -> (w280:cluster{dbl[], dbl[]}[])
                        n232 = for {
                          tunnel: [w283] -> w281 mode=indexing
                          tunnel: w280 -> [w282] mode=indexing
                          i -> [w284]
                          n233 = case shown="0" w284 {
                            tunnel: [w285 w287] -> w283
                            tunnel: w282 -> [w285 _]
                            frame Default {
                            }
                            frame 0 {
                              n234 = global read "Global.vi" "左工位判定框"() -> (w293:T6)
                              n235 = Unbundle By Name(w293) -> ("X.下限"=w290:dbl, "X.上限"=w286:dbl, "Y.下限"=w291:dbl, "Y.上限"=w292:dbl)
                              n236 = Build Array(w286, w286, w290, w290, w286) -> (w288:dbl[])
                              n237 = Build Array(w291, w292, w292, w291, w291) -> (w289:dbl[])
                              n238 = Bundle(w288, w289) -> (w287:cluster{dbl[], dbl[]})  [unwired: 1 in]
                            }
                          }
                        }
                        n239 = local write "左工位曲线"(w281) -> ()
                      }
                    }
                  }
                  frame "右工位" {
                    n240 = stacked-sequence {
                      frame #0 {
                        n241 = for {
                          N: 50 -> [_]
                          tunnel: [cluster{dbl[], dbl[]} {[], []}] -> w294 mode=indexing
                        }
                        n242 = local write "右工位曲线"(w294) -> ()
                      }
                      frame #1 {
                        n243 = local read "右工位曲线"() -> (w297:cluster{dbl[], dbl[]}[])
                        n244 = for {
                          tunnel: [w300] -> w298 mode=indexing
                          tunnel: w297 -> [w299] mode=indexing
                          i -> [w301]
                          n245 = case shown="0" w301 {
                            tunnel: [w302 w304] -> w300
                            tunnel: w299 -> [w302 _]
                            frame Default {
                            }
                            frame 0 {
                              n246 = global read "Global.vi" "右工位判定框"() -> (w310:T6)
                              n247 = Unbundle By Name(w310) -> ("X.下限"=w307:dbl, "X.上限"=w303:dbl, "Y.下限"=w308:dbl, "Y.上限"=w309:dbl)
                              n248 = Build Array(w303, w303, w307, w307, w303) -> (w305:dbl[])
                              n249 = Build Array(w308, w309, w309, w308, w308) -> (w306:dbl[])
                              n250 = Bundle(w305, w306) -> (w304:cluster{dbl[], dbl[]})  [unwired: 1 in]
                            }
                          }
                        }
                        n251 = local write "右工位曲线"(w298) -> ()
                      }
                    }
                  }
                }
              }
              frame 1000 {
                n252 = global read "Global.vi" "上序状态"() -> (w313:refnum<vi>)
                n253 = property class="Str"(reference=w313, "Text.Text"="" ("文本.文本"), "Text.BGColor"=u32 16777216 ("文本.文本颜色:背景色")) -> ()  [unwired: 1 in, 2 out]
                n254 = local write "STEP"("扫码" ("STEP")) -> ()
                n255 = call "备用1.vi"("枚举"=enum16{"Read", "Write"}."Write", "Status_Write"=u16 1001 ("备用1")) -> ()  [unwired: 9 in, 1 out]
              }
              frame 1001 {
              }
            }
          }
          frame "报表" {
            n256 = stacked-sequence {
              seq-local: [w321 _ _] -> [_ w323 _]
              frame #0 {
                n257 = call "备用1.vi"("枚举"=enum16{"Read", "Write"}."Write", "Status_Write"=u16 0 ("备用1")) -> ()  [unwired: 9 in, 1 out]
                n258 = global read "Global.vi" "追溯码"() -> (w319:string)
                n259 = call "Report_A131258.vi"("文件重命名"=TRUE, "文件名称"=w319, "布尔数组"="判定结果") -> ("工件状态"=w321:string)  [unwired: 7 in, 1 out]
              }
              frame #1 {
                n260 = global read "Global1.vi" "联机模式"() -> (w324:enum16{"单机", "追溯"})
                n261 = case shown="\"追溯\"" w324 {
                  tunnel: w323 -> [_ w325]
                  frame "单机", Default {
                  }
                  frame "追溯" {
                    n262 = global read "Global.vi" "Result"() -> (w330:refnum<vi>)
                    n263 = property class="Tbl"(reference=w330) -> (reference out=w335:refnum<vi>, error out=w332:errorcluster, "Row Headers[]"=w333:string[])  [unwired: 1 in]
                    n264 = property class="Tbl"(reference=w335, error in=w332) -> (error out=w331:errorcluster, "Value"=w334:string[][])  [unwired: 1 out]
                    n265 = for {
                      tunnel: w334 -> [w339] mode=indexing
                      tunnel: w333 -> [w340] mode=indexing
                      tunnel: [w337] -> w329 mode=indexing if=w338
                      shift-right: [w336] -> _
                      shift-left: w331 -> [w336]
                      n266 = Build Array (concatenate)(w340, w339) -> (w337:string[])
                      n267 = Index Array(array=w339) -> (element=w341:string)  [unwired: 1 in]
                      n268 = case shown="默认" w341 {
                        tunnel: [TRUE FALSE] -> w338
                        frame Default {
                        }
                        frame "" {
                        }
                      }
                    }
                    n269 = global read "Global.vi" "DEVICED_ID"() -> (w328:string)
                    n270 = global read "Global.vi" "CODE_ID"() -> (w327:string)
                    n271 = global read "Global.vi" "USER_ID"() -> (w326:string)
                    n272 = call "UPTEST.vi"("Result"=w329, "CODE_ID"=w327, "DEVICE_ID"=w328) -> ()  [unwired: 6 in, 1 out]
                    n273 = call "UPRESULT.vi"("DEVICE_ID"=w328, "USER_ID"=w326, "CODE_ID"=w327, "RESULT_VALUE"=w325) -> ()  [unwired: 11 in, 1 out]
                  }
                }
              }
              frame #2 {
                n274 = local write "STEP"("等待" ("STEP")) -> ()
                n275 = global write "Global.vi" "当前试验项"(enum16{"左工位", "右工位", "完成"}."左工位" ("当前试验项")) -> ()
              }
            }
          }
        }
        n276 = global read "Global.vi" "程序关闭"() -> (w18:bool)
      }
      n277 = while {
        shift-right: [w347] -> w15
        shift-left: w14 -> [w348]
        stop <- w349 stop-if-true
        n278 = Wait Until Next ms Multiple(millisecond multiple=u32 10 ("毫秒倍数")) -> ()  [unwired: 1 out]
        n279 = event shown="[4] \"左工位曲线\", \"右工位曲线\": 标尺范围更改" {
          selector: w348 -> [_ _ _ _ _ _ _ _]
          dyn-events: [_ _ _ _ _ _ _ _] -> w347
          timeout: 100 -> [_ _ _ _ _ _ _ _]
          event Timeout {
            n280 = event-data() -> ()  [unwired: 1 in, 3 out]
            n281 = disable-structure shown="禁用" {
              frame Disabled {
                n282 = call "Obtain Broadcast Events for Registration.vi"() -> ("Already running?"=w351:bool)  [unwired: 9 in, 2 out]
                n283 = case shown="真" w351 {
                  frame False {
                    n284 = local write "STEP"("手动" ("STEP")) -> ()
                  }
                  frame True {
                    n285 = call "错误代码.vi"() -> ("Status_Read"=w353:u32)  [unwired: 11 in]
                    n286 = feedback #1() -> (w363:u32)  [unwired: 1 in]
                    n287 = feedback-in #1(w353) -> ()
                    n288 = case shown="0" w353 {
                      frame 0 {
                        n289 = global read "Global.vi" "报警图标"() -> (w364:refnum<vi>)
                        n290 = property class="Bool"(reference=w364, "Visible"=FALSE ("可见")) -> ()  [unwired: 1 in, 2 out]
                      }
                      frame 1, Default {
                        n291 = global read "Global.vi" "报警图标"() -> (w367:refnum<vi>)
                        n292 = property class="Bool"(reference=w367, "Visible"=TRUE ("可见")) -> ()  [unwired: 1 in, 2 out]
                      }
                    }
                    n293 = Greater Or Equal?(x=w353, y=i16 5000) -> (x >= y?=w361:bool)
                    n294 = Less?(x=w353, y=i16 5200) -> (x < y?=w362:bool)
                    n295 = Equal?(x=w353, y=w363) -> (x = y?=w360:bool)
                    n296 = global read "Global.vi" "报警图标"() -> (w355:refnum<vi>)
                    n297 = And(x=w361, y=w362) -> (x .and. y?=w354:bool)
                    n298 = property class="Bool"(reference=w355, "Value"=w354) -> ()  [unwired: 1 in, 2 out]
                    n299 = Bundle By Name(cluster=errorcluster {"status"=FALSE, "code"=0, "source"=""} ("错误常量"), "status"=w354, "code"=w353) -> (w359:errorcluster)
                    n300 = case shown="假" w360 {
                      tunnel: w359 -> [w368 _]
                      frame False {
                        n301 = call "报警处理.vi"("错误常量"=w368) -> ()  [unwired: 9 in, 2 out]
                      }
                      frame True {
                      }
                    }
                  }
                }
              }
              frame Enabled {
              }
            }
          }
          event User Event {
            n302 = event-data() -> ("产品标尺"=w369:string)  [unwired: 1 in, 4 out]
            n303 = control-ref of="管柱保持力试验"() -> (w374:refnum<vi>)
            n304 = control-ref of="左工位曲线"() -> (w370:refnum<vi>)
            n305 = control-ref of="锁紧/开启"() -> (w373:refnum<vi>)
            n306 = control-ref of="右工位曲线"() -> (w372:refnum<vi>)
            n307 = control-ref of="角度调节力试验"() -> (w375:refnum<vi>)
            n308 = Build Array(w374, w372, w373, w375, w370) -> (w371:refnum<vi>[])
            n309 = for {
              tunnel: w371 -> [w377] mode=indexing
              tunnel: w369 -> [w376]
              n310 = call "XY_conf.vi"("方式"=enum16{"写入", "读取"}."读取", "产品"=w376, "XY图引用"=w377) -> ()  [unwired: 4 in, 1 out]
            }
          }
          event User Event {
            n311 = event-data() -> ("试验项"=→"试验项目":T1)  [unwired: 1 in]
            n312 = disable-structure shown="禁用" {
              frame Disabled {
                n313 = local read "管柱保持力试验"() -> (w383:cluster{dbl[], dbl[]}[])
                n314 = global read "判定参数.vi" "最大位移"() -> (w380:dbl)
                n315 = global read "判定参数.vi" "最大拉力"() -> (w382:dbl)
                n316 = global read "判定参数.vi" "最小拉力"() -> (w381:dbl)
                n317 = for {
                  tunnel: [w390] -> w384 mode=indexing
                  tunnel: w383 -> [w389] mode=indexing
                  tunnel: w382 -> [w388]
                  tunnel: w381 -> [w387]
                  tunnel: w380 -> [w386]
                  tunnel: w380 -> [w385]
                  i -> [w391]
                  n318 = case shown="1" w391 {
                    tunnel: [w392 w393] -> w390
                    tunnel: w389 -> [w392 _]
                    tunnel: w388 -> [_ w397]
                    tunnel: w387 -> [_ w396]
                    tunnel: w386 -> [_ w395]
                    tunnel: w385 -> [_ w394]
                    frame 0, Default {
                    }
                    frame 1 {
                      n319 = Build Array(w395, w395, w394, w394, w395) -> (w399:dbl[])
                      n320 = Build Array(w396, w397, w397, w396, w396) -> (w398:dbl[])
                      n321 = Bundle(w399, w398) -> (w393:cluster{dbl[], dbl[]})  [unwired: 1 in]
                    }
                  }
                }
                n322 = local write "管柱保持力试验"(w384) -> ()
              }
              frame Enabled {
              }
            }
            n323 = disable-structure shown="禁用" {
              disable-tunnel: _ -> [w400 _]
              frame Disabled {
                n324 = global read "A180648.vi" "检测结果"() -> (w403:string[][][])
                n325 = global read "Global.vi" "Result"() -> (w401:refnum<vi>)
                n326 = Index Array(array=w403, index (dim 0)=w400) -> (element=w402:string[][])  [unwired: 2 in]
                n327 = property class="Tbl"(reference=w401, "Value"=w402) -> ()  [unwired: 1 in, 2 out]
              }
              frame Enabled {
              }
            }
          }
          event "试验项目": Value Change {
            n328 = event-data() -> ("NewVal"=w404:T1)  [unwired: 1 in]
            n329 = disable-structure shown="禁用" {
              disable-tunnel: w404 -> [w408 _]
              frame Disabled {
                n330 = global read "A180648.vi" "检测结果"() -> (w407:string[][][])
                n331 = global read "Global.vi" "Result"() -> (w405:refnum<vi>)
                n332 = Index Array(array=w407, index (dim 0)=w408) -> (element=w406:string[][])  [unwired: 2 in]
                n333 = property class="Tbl"(reference=w405, "Value"=w406) -> ()  [unwired: 1 in, 2 out]
              }
              frame Enabled {
              }
            }
          }
          event "左工位曲线", "右工位曲线": Scale Range Change {
            n334 = event-data() -> ("CtlRef"=w411:refnum<vi>)  [unwired: 1 in, 4 out]
            n335 = global read "Global.vi" "产品型号"() -> (w409:string)
            n336 = call "XY_conf.vi"("方式"=enum16{"写入", "读取"}."写入", "产品"=w409, "XY图引用"=w411) -> ()  [unwired: 4 in, 1 out]
          }
          event Panel Close {
            n337 = event-data() -> ()  [unwired: 1 in, 4 out]
            n338 = global write "Global.vi" "程序关闭"(TRUE ("程序关闭")) -> ()
          }
          event "管柱保持力试验", "锁紧/开启", "角度调节力试验", "振动1NVH-FFT", "左工位曲线", "右工位曲线", "逆向空载试验": Mouse Enter; "管柱保持力试验", "锁紧/开启", "角度调节力试验", "振动1NVH-FFT", "左工位曲线", "右工位曲线", "逆向空载试验": Mouse Leave; "管柱保持力试验", "锁紧/开启", "角度调节力试验", "振动1NVH-FFT", "左工位曲线", "右工位曲线", "逆向空载试验": Cursor Move {
            n339 = event-data() -> ("CtlRef"=w415:refnum<vi>, "Type"=w413:T7)  [unwired: 1 in]
            n340 = call "CursorShow.vi"("nameShow"=TRUE, "Type"=w413, "Graph"=w415) -> ()  [unwired: 7 in, 2 out]
          }
          event "管柱保持力试验", "锁紧/开启", "角度调节力试验", "振动1NVH-FFT", "左工位曲线", "右工位曲线", "逆向空载试验": Mouse Down {
            n341 = event-data() -> ("CtlRef"=w420:refnum<vi>, "Coords"=w419:T8, "Type"=w417:T7)  [unwired: 1 in]
            n342 = invoke class="WFGraph" method="Map Coords To XY"(reference=w420, "Coords"=w419) -> (reference out=w418:refnum<vi>, "XY"=w416:cluster{"X":dbl, "Y":dbl})  [unwired: 5 in, 5 out]
            n343 = call "CursorShow.vi"("游标.游标位置"=w416, "Type"=w417, "Graph"=w418) -> ()  [unwired: 7 in, 2 out]
          }
        }
        n344 = global read "Global.vi" "程序关闭"() -> (w349:bool)
      }
    }
  }
  n345 = Unregister For Events(event registration refnum=w6) -> ()  [unwired: 1 in, 1 out]
  n346 = disable-structure shown="禁用" {
    frame Disabled {
      n347 = stacked-sequence {
        frame #0 {
          w423 = "请扫码！" ("提示信息")
          n348 = call "输入框.vi"("提示信息"=w423) -> ("条形码输出"=w421:string)
          n349 = call "浮动通知.vi"("通知内容"=w423) -> ()  [unwired: 11 in]
          n350 = case shown="默认" w421 {
            selector: w421 -> [w425 _]
            tunnel: [w426 "退出自动" ("State(s) in Front (\"\")")] -> w422
            frame Default {
              n351 = global read "Global1.vi" "联机模式"() -> (w424:enum16{"单机", "追溯"})
              n352 = case shown="\"追溯\"" w424 {
                tunnel: ["初始化" ("State(s) in Front (\"\")") w434] -> w426
                tunnel: w425 -> [_ w432]
                frame "单机", Default {
                  n353 = shared-variable "我的电脑\\180压装.lvlib\\备用1"(u16 1002 ("备用1")) -> ()  [unwired: 1 in, 1 out]
                }
                frame "追溯" {
                  n354 = call "Get_CODE_ID.vi"("CODE_MAIN"=w432) -> ("CODE_ID"=w430:string)  [unwired: 10 in]
                  n355 = global read "Global.vi" "PRODUCT_ID"() -> (w429:string)
                  n356 = global write "Global.vi" "CODE_ID"(w430) -> ()
                  n357 = call "GET_PRESTATUS.vi"("CODE_ID"=w430, "PRODUCT_ID"=w429) -> ("字符串"=w431:string, "OK?"=w433:bool)  [unwired: 8 in]
                  n358 = case shown="真" w433 {
                    tunnel: [w436 "初始化" ("State(s) in Front (\"\")")] -> w434
                    tunnel: w431 -> [w435 _]
                    frame False {
                      n359 = case shown="默认" w435 {
                        tunnel: ["扫码" ("State(s) in Front (\"\")") "扫码" ("State(s) in Front (\"\")")] -> w436
                        frame Default {
                          n360 = global read "Global.vi" "上序状态"() -> (w437:refnum<vi>)
                          n361 = property class="Str"(reference=w437, "Text.BGColor"=u32 16776960 ("文本.文本颜色:背景色")) -> (reference out=w439:refnum<vi>)  [unwired: 1 in, 1 out]
                          n362 = One Button Dialog(message="前序检测漏序！" ("消息")) -> ()  [unwired: 1 in, 1 out]
                          n363 = property class="Str"(reference=w439, "Value"="上序漏序" ("上序状态")) -> ()  [unwired: 1 in, 2 out]
                        }
                        frame "NG" {
                          w444 = "前序检测不合格！" ("消息")
                          n364 = global read "Global.vi" "上序状态"() -> (w443:refnum<vi>)
                          n365 = property class="Str"(reference=w443, "Text.BGColor"=u32 16711680 ("文本.文本颜色:背景色")) -> (reference out=w446:refnum<vi>, error out=w445:errorcluster)  [unwired: 1 in]
                          n366 = One Button Dialog(message=w444) -> ()  [unwired: 1 in, 1 out]
                          n367 = property class="Str"(reference=w446, error in=w445, "Value"=w444) -> ()  [unwired: 2 out]
                        }
                      }
                    }
                    frame True {
                      n368 = global read "Global.vi" "上序状态"() -> (w450:refnum<vi>)
                      n369 = global read "Global.vi" "生产数量"() -> (w455:i32)
                      n370 = property class="Str"(reference=w450, "Text.BGColor"=u32 6618880 ("文本.文本颜色:背景色")) -> (reference out=w453:refnum<vi>, error out=w452:errorcluster)  [unwired: 1 in]
                      n371 = Increment(x=w455) -> (x+1=w456:i32)
                      n372 = global write "Global.vi" "生产数量"(w456) -> ()
                      n373 = shared-variable "我的电脑\\180压装.lvlib\\备用1"(u16 1002 ("备用1")) -> ()  [unwired: 1 in, 1 out]
                      n374 = property class="Str"(reference=w453, error in=w452, "Value"="合格" ("上序状态")) -> ()  [unwired: 2 out]
                    }
                  }
                }
              }
            }
            frame "", "exit" {
            }
          }
          n375 = global write "Global.vi" "追溯码"(w421) -> ()
          n376 = local write "STEP"(w422) -> ()
        }
        frame #1 {
          n377 = Wait (ms)(milliseconds to wait=u32 100 ("等待时间（毫秒）")) -> ()  [unwired: 1 out]
        }
      }
    }
    frame Enabled {
    }
  }
